vi "Time Update INI File.vi"(8 "error in (no error)":errorcluster) -> (0 "error out":errorcluster)   [LabVIEW 2011]
uses:
  <vilib>/Utility/config.llb/NI_LVConfig.lvlib
  <vilib>/Utility/config.llb/Write Key (String).vi
  server/database/Templates/Template Record.ctl
  ITK EXT/utils/strutil.llb/Case Matching.ctl
panel:
  out "Status":string
  out "Template Dir":path
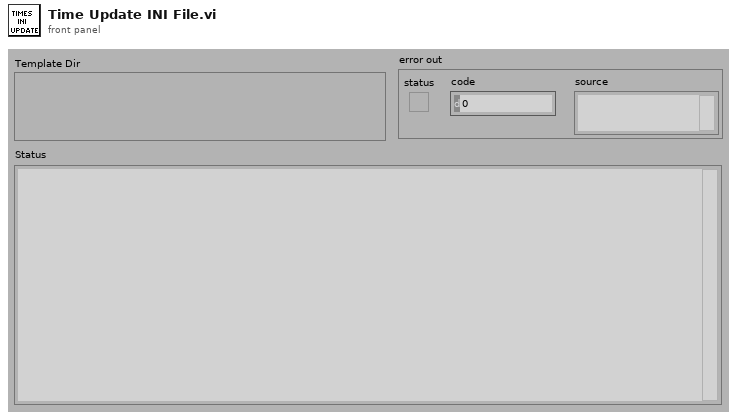
[diagram p1: front panel]
types:
  T1 = typedef "Template Record.ctl" = cluster{"ixTemplate":i32, "sxTemplateId":string, "sDescription":string, "sCreator":string, "tCreationDate":timestamp, "sModifier":string, "tModifiedDate":timestamp, "sType":string, "sStyle":string, "sFormat":string, "dWidth":dbl, "dHeight":dbl, "sFilename":string, "sScript":string, "sLayout":string, "sEditor":string, "sStyleProcess":string}
  T2 = enum32{"invalid app kind", "Development System", "Run Time System", "Student Edition", "Embedded LabVIEW", "Evaluation", "Custom"}
  T3 = typedef "Case Matching.ctl" = enum16{"a != A", "a == A", "system"}
  T4 = typedef "Keyed Array.ctl" = cluster{"keys":string[], "values":string[]}
  T5 = typedef "NI_LVConfig.lvlib/Config Data RefNum.ctl" = refnum<k1>
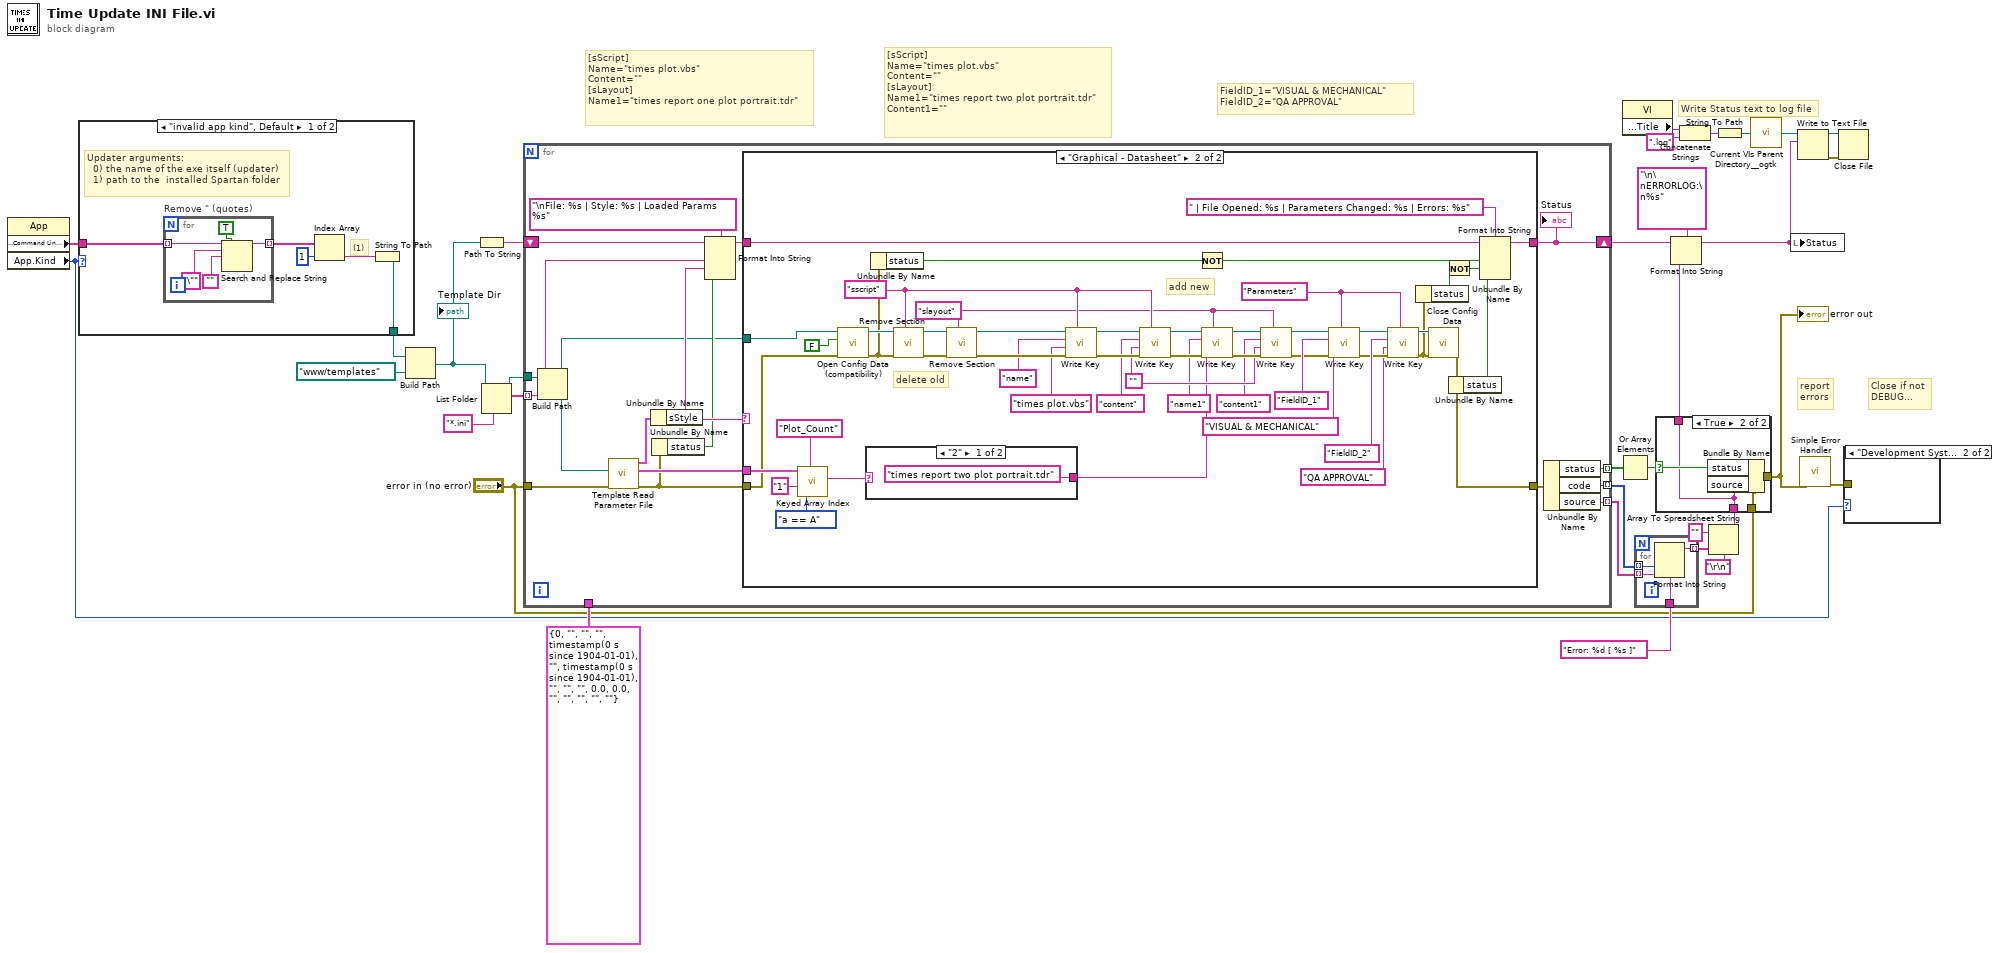
[diagram p0: block diagram]
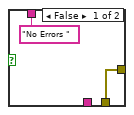
[diagram p2: hidden frame]
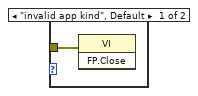
[diagram p3: hidden frame]
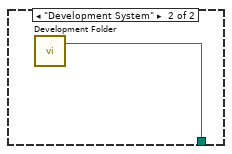
[diagram p4: hidden frame]
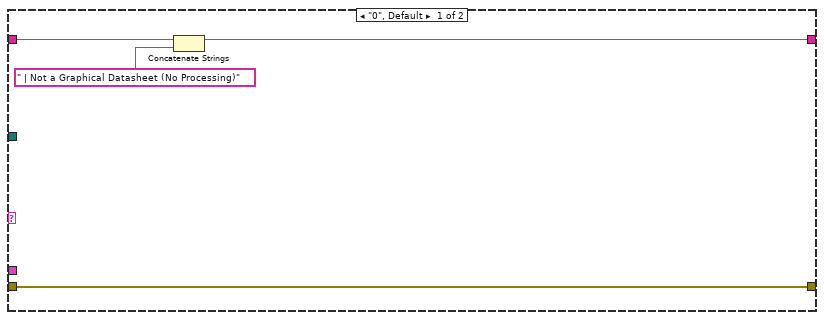
[diagram p5: hidden frame]
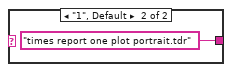
[diagram p6: hidden frame]
diagram:
  # "Write Status text to log file"
  # "FieldID_1=\"VISUAL & MECHANICAL\"\nFieldID_2=\"QA APPROVAL\""
  # "report\nerrors"
  # "Close if not\nDEBUG..."
  # "[sScript]\nName=\"times plot.vbs\"\nContent=\"\"\n[sLayout]\nName1=\"times report two plot portrait.tdr\"\nContent1=\"\""
  # "[sScript]\nName=\"times plot.vbs\"\nContent=\"\"\n[sLayout]\nName1=\"times report one plot portrait.tdr\""
  n1 = property class="App"() -> ("Application:Command Line Arguments"=w32:string[], "App.Kind"=w6:T2)  [unwired: 2 in, 2 out]
  n2 = case shown="\"invalid app kind\", Default" w6 {
    tunnel: w32 -> [w38 _]
    tunnel: [w34 w44] -> w30
    frame "invalid app kind", Default {
      # "(1)"
      # "Updater arguments:\n  0) the name of the exe itself (updater)\n  1) path to the  installed Spartan folder"
      n3 = for "Remove \" (quotes)" {
        tunnel: w38 -> [w41] mode=indexing
        tunnel: [w40] -> w36 mode=indexing
        n4 = Search and Replace String(replace all?=TRUE, input string=w41, search string="\"", replace string="") -> (result string=w40:string)  [unwired: 1 in, 6 out]
      }
      n5 = Index Array(array=w36, index=1) -> (element=w35:string)
      n6 = String To Path(string=w35) -> (path=w34:path)
    }
    frame "Development System" {
      n7 = call "Development Folder.vi"() -> ("Development Folder"=w44:path)  [unwired: 1 out]
    }
  }
  n8 = Build Path(base path=w30, name or relative path=path "www/templates" ("stripped path")) -> (appended path=w24:path)
  "Template Dir" <- w24
  n9 = Path To String(path=w24) -> (string=w25:string)
  n10 = List Folder(path=w24, pattern="*.ini") -> (path out=w27:path, filenames=w26:string[])  [unwired: 1 in, 3 out]
  n11 = for {
    tunnel: w27 -> [w61]
    tunnel: w26 -> [w55] mode=indexing
    tunnel: T1 {"ixTemplate"=0, "sxTemplateId"="", "sDescription"="", "sCreator"="", "tCreationDate"=timestamp(0 s since 1904-01-01), "sModifier"="", "tModifiedDate"=timestamp(0 s since 1904-01-01), "sType"="", "sStyle"="", "sFormat"="", "dWidth"=0.0, "dHeight"=0.0, "sFilename"="", "sScript"="", "sLayout"="", "sEditor"="", "sStyleProcess"=""} ("Template Record") -> [_]
    shift-right: [w50] -> w13
    shift-left: w25 -> [w56]
    tunnel: "error in (no error)" -> [w60]
    tunnel: [w47] -> w23 mode=indexing
    tunnel: [w46] -> w21 mode=indexing
    tunnel: [w45] -> w20 mode=indexing
    n12 = Build Path(base path=w61, name or relative path=w55) -> (appended path=w49:path)
    n13 = call "Template Read Parameter File.vi"("error in (no error)"=w60, "Alternate Path (\"\")"=w49) -> ("error out"=w53:errorcluster, "Parameters"=w58:T4, "updated Template Record"=w59:T1)  [unwired: 1 in, 6 out]
    n14 = Unbundle By Name(w59) -> ("sStyle"=w54:string)
    n15 = Unbundle By Name(w53) -> ("status"=w52:bool)
    n16 = Format Into String(format string="\nFile: %s | Style: %s | Loaded Params %s", initial string=w56, w55, w54, w52) -> (resulting string=w51:string)  [unwired: 1 in, 1 out]
    n17 = case shown="\"Graphical - Datasheet\"" w54 {
      tunnel: w53 -> [w65 w109]
      tunnel: [w65 w69] -> w48
      tunnel: w58 -> [_ w111]
      tunnel: w49 -> [_ w108]
      tunnel: w51 -> [w63 w75]
      tunnel: [w62 w74] -> w50
      frame "0", Default {
        n18 = Concatenate Strings(w63, " | Not a Graphical Datasheet (No Processing)" ("format string")) -> (w62:string)
      }
      frame "Graphical - Datasheet" {
        w77 = "Parameters" ("section")
        w90 = ""
        w92 = "slayout" ("section")
        w93 = "sscript" ("section")
        # "add new"
        # "delete old"
        n19 = call "Keyed Array Index.vi"("case matching (sensitive)"=Case_Matching."a == A", "default value"="1", "key"="Plot_Count" ("format string"), "array in"=w111) -> ("value"=w110:string)  [unwired: 3 out]
        n20 = call <vilib>:"Open Config Data (compatibility).vi"("error in (no error)"=w109, "create file if necessary (T)"=FALSE ("create file if necessary? (T)"), "configuration file path"=w108) -> ("error out"=w73:errorcluster, "refnum"=w106:T5)  [unwired: 6 in, 1 out]
        n21 = case shown="\"2\"" w110 {
          tunnel: ["times report two plot portrait.tdr" "times report one plot portrait.tdr"] -> w88
          frame "2" {
          }
          frame "1", Default {
          }
        }
        n22 = Unbundle By Name(w73) -> ("status"=w72:bool)
        n23 = call <vilib>:"Remove Section.vi"("section"=w93, "error in (no error)"=w73, "refnum"=w106) -> ("error out"=w105:errorcluster, "refnum out"=w104:T5)  [unwired: 7 out]
        n24 = call <vilib>:"Remove Section.vi"("section"=w92, "error in (no error)"=w105, "refnum"=w104) -> ("error out"=w97:errorcluster, "refnum out"=w96:T5)  [unwired: 7 out]
        n25 = call-poly <vilib>:"Write Key.vi"("section"=w93, "error in (no error)"=w97, "value"="times plot.vbs", "key"="name", "refnum"=w96) -> ("error out"=w98:errorcluster, "refnum out"=w99:T5)  [unwired: 1 in, 4 out]
        n26 = call-poly <vilib>:"Write Key.vi"("section"=w93, "error in (no error)"=w98, "value"=w90, "key"="content", "refnum"=w99) -> ("error out"=w100:errorcluster, "refnum out"=w101:T5)  [unwired: 1 in, 4 out]
        n27 = Not(x=w72) -> (.not. x?=w67:bool)
        n28 = call-poly <vilib>:"Write Key.vi"("section"=w92, "error in (no error)"=w100, "value"=w88, "key"="name1", "refnum"=w101) -> ("error out"=w103:errorcluster, "refnum out"=w102:T5)  [unwired: 1 in, 4 out]
        n29 = call-poly <vilib>:"Write Key.vi"("section"=w92, "error in (no error)"=w103, "value"=w90, "key"="content1", "refnum"=w102) -> ("error out"=w81:errorcluster, "refnum out"=w82:T5)  [unwired: 1 in, 4 out]
        n30 = call-poly <vilib>:"Write Key.vi"("section"=w77, "error in (no error)"=w81, "value"="VISUAL & MECHANICAL", "key"="FieldID_1", "refnum"=w82) -> ("error out"=w83:errorcluster, "refnum out"=w84:T5)  [unwired: 1 in, 4 out]
        n31 = call-poly <vilib>:"Write Key.vi"("section"=w77, "error in (no error)"=w83, "value"="QA APPROVAL", "key"="FieldID_2", "refnum"=w84) -> ("error out"=w71:errorcluster, "refnum out"=w80:T5)  [unwired: 1 in, 4 out]
        n32 = Unbundle By Name(w71) -> ("status"=w70:bool)
        n33 = call <vilib>:"Close Config Data.vi"("error in (no error)"=w71, "refnum"=w80) -> ("error out"=w69:errorcluster)  [unwired: 1 in, 8 out]
        n34 = Not(x=w70) -> (.not. x?=w66:bool)
        n35 = Unbundle By Name(w69) -> ("status"=w68:bool)
        n36 = Format Into String(format string=" | File Opened: %s | Parameters Changed: %s | Errors: %s", initial string=w75, w67, w66, w68) -> (resulting string=w74:string)  [unwired: 1 in, 1 out]
      }
    }
    "Status" <- w50
    n37 = Unbundle By Name(w48) -> ("status"=w47:bool, "code"=w46:i32, "source"=w45:string)
  }
  n38 = Or Array Elements(Boolean array=w23) -> (logical OR=w5:bool)
  n39 = property class="VI"() -> ("Front Panel.Title"=w3:string)  [unwired: 2 in, 2 out]
  n40 = for {
    tunnel: "Error: %d [ %s ]" ("format string") -> [w120]
    tunnel: w21 -> [w119] mode=indexing
    tunnel: w20 -> [w118] mode=indexing
    tunnel: [w117] -> w19 mode=indexing
    n41 = Format Into String(format string=w120, w119, w118) -> (resulting string=w117:string)  [unwired: 2 in, 1 out]
  }
  n42 = Concatenate Strings(w3, ".log" ("new ending (none)")) -> (w1:string)
  n43 = Array To Spreadsheet String(delimiter (Tab)="\r\n", array=w19, 3:"" ("format string")) -> (spreadsheet string=w12:string)
  n44 = case shown="True" w5 {
    selector: w5 -> [_ w124]
    tunnel: [w122 w126] -> w16
    tunnel: "error in (no error)" -> [w122 w125]
    tunnel: w12 -> [_ w123]
    tunnel: ["No Errors " ("spreadsheet string") w123] -> w4
    frame False {
    }
    frame True {
      n45 = Bundle By Name(cluster=w125, "status"=w124, "source"=w123) -> (w126:errorcluster)
    }
  }
  "error out" <- w16
  n46 = Format Into String(format string="\n\nERRORLOG:\n%s", initial string=w13, w4) -> (resulting string=w9:string)  [unwired: 1 in, 1 out]
  n47 = String To Path(string=w1) -> (path=w11:path)
  n48 = call "Current VIs Parent Directory__ogtk.vi"("Relative path (.)"=w11) -> ("Parent Directory (+ Relative)"=w10:path)  [unwired: 4 out]
  n49 = local write "Status"(w9) -> ()
  n50 = Write to Text File(file (use dialog)=w10, text=w9) -> (refnum out=w7:refnum<file>, error out=w8:errorcluster)  [unwired: 1 in, 2 out]
  n51 = call <vilib>:"Simple Error Handler.vi"("error in (no error)"=w16) -> ("error out"=w29:errorcluster)  [unwired: 1 in, 7 out]
  n52 = Close File(refnum=w7, error in=w8) -> ()  [unwired: 2 out]
  n53 = case shown="\"Development System\"" w6 {
    tunnel: w29 -> [w127 _]
    frame "invalid app kind", Default {
      n54 = invoke class="VI" method="FP.Close"(error in=w127) -> ()  [unwired: 2 in, 3 out]
    }
    frame "Development System" {
    }
  }
